vi "Compare Hits With Coinchuntlim.vi"(1 "Type":T1(ring), 2 "Make check":bool) -> (0 "Perform coinc hunt?":bool)   [LabVIEW 2016]
uses:
  Global Variables/Coincidence hunt limit.vi
  Global Variables/Scintillator IDs.vi
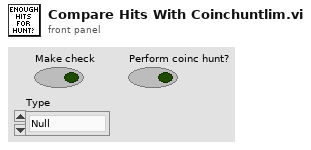
[diagram p1: front panel]
types:
  T1 = enum16{"Null", "BottomLayer", "TopAndBottom", "TopLayer"}
  T2 = enum16{"InsertHits", "GetHits", "GetHitsDestructive", "GetNumOfHits"}
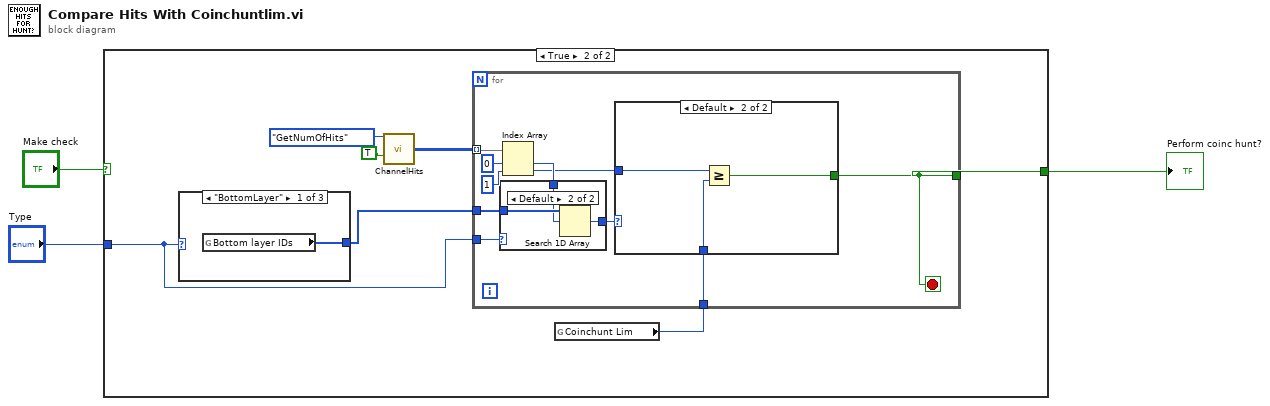
[diagram p0: block diagram]
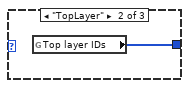
[diagram p3: hidden frame]
diagram:
  n1 = case shown="True" "Make check" {
    tunnel: [_ w9] -> w3
    tunnel: "Type" -> [_ w4]
    frame False {
    }
    frame True {
      n2 = case shown="\"BottomLayer\"" w4 {
        tunnel: [w11 w12 _] -> w5
        frame "BottomLayer" {
          n3 = global read "Scintillator IDs.vi" "Bottom layer IDs"() -> (w11:i8[])
        }
        frame "TopLayer" {
          n4 = global read "Scintillator IDs.vi" "Top layer IDs"() -> (w12:i8[])
        }
        frame "TopAndBottom", Default {
        }
      }
      n5 = call "ChannelHits.vi"("Action"=T2."GetNumOfHits", "Assert Semaphore"=TRUE) -> ("NumOfHits all channels"=w6:i32[][])  [unwired: 6 in, 7 out]
      n6 = global read "Coincidence hunt limit.vi" "Coinchunt Lim"() -> (w8:i32)
      n7 = for {
        tunnel: w6 -> [w21] mode=indexing
        tunnel: w8 -> [w22]
        tunnel: [w14] -> w9
        tunnel: w5 -> [w18]
        tunnel: w4 -> [w13]
        stop <- w14 stop-if-true
        n8 = Index Array(array=w21, index #1=0 ("index"), index #2=1 ("index")) -> (element #1=w17:i32, element #2=w15:i32)
        n9 = case shown="Default" w13 {
          tunnel: w18 -> [_ w25]
          tunnel: w17 -> [_ w24]
          tunnel: [_ w23] -> w16
          frame "TopAndBottom" {
          }
          frame Default {
            n10 = Search 1D Array(1D array=w25, element=w24) -> (index of element=w23:i32)  [unwired: 1 in]
          }
        }
        n11 = case shown="Default" w16 {
          tunnel: w22 -> [_ w28]
          tunnel: [_ w27] -> w14
          tunnel: w15 -> [_ w26]
          frame -1 {
          }
          frame Default {
            n12 = Greater Or Equal?(x=w26, y=w28) -> (x >= y?=w27:bool)
          }
        }
      }
    }
  }
  "Perform coinc hunt?" <- w3
